vi "sum values per sequence.vi"(8 "error in":errorcluster, 11 "cycle results cluster IN":T1) -> (0 "Sequence Results":dbl[][](array[numeric]), 3 "cycle results cluster out":T1)   [LabVIEW 2016]
doc: "Takes a sample type and sorts by sequence"
uses:
  controls/cycle results control.ctl
  <vilib>/Analysis/baseanly.llb/Mean (DBL).vi
  <vilib>/Analysis/NI_AALBase.lvlib
panel:
  out "error out":errorcluster
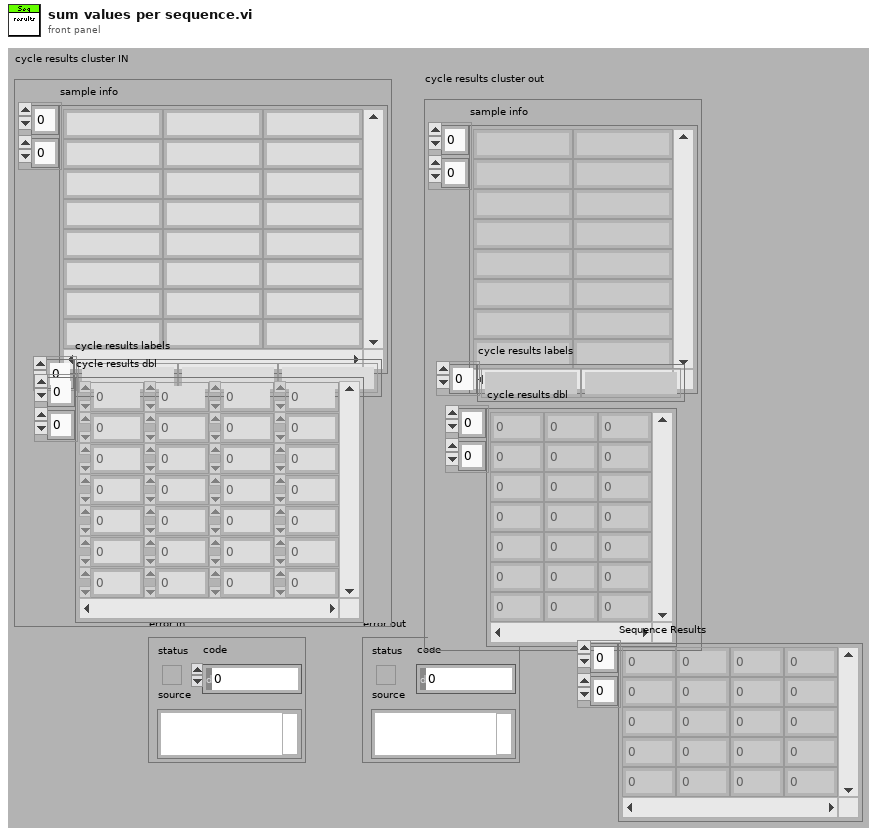
[diagram p1: front panel]
types:
  T1 = typedef "cycle results control.ctl" = cluster{"sample info":string[][], "cycle results labels":string[], "cycle results dbl":dbl[][]}
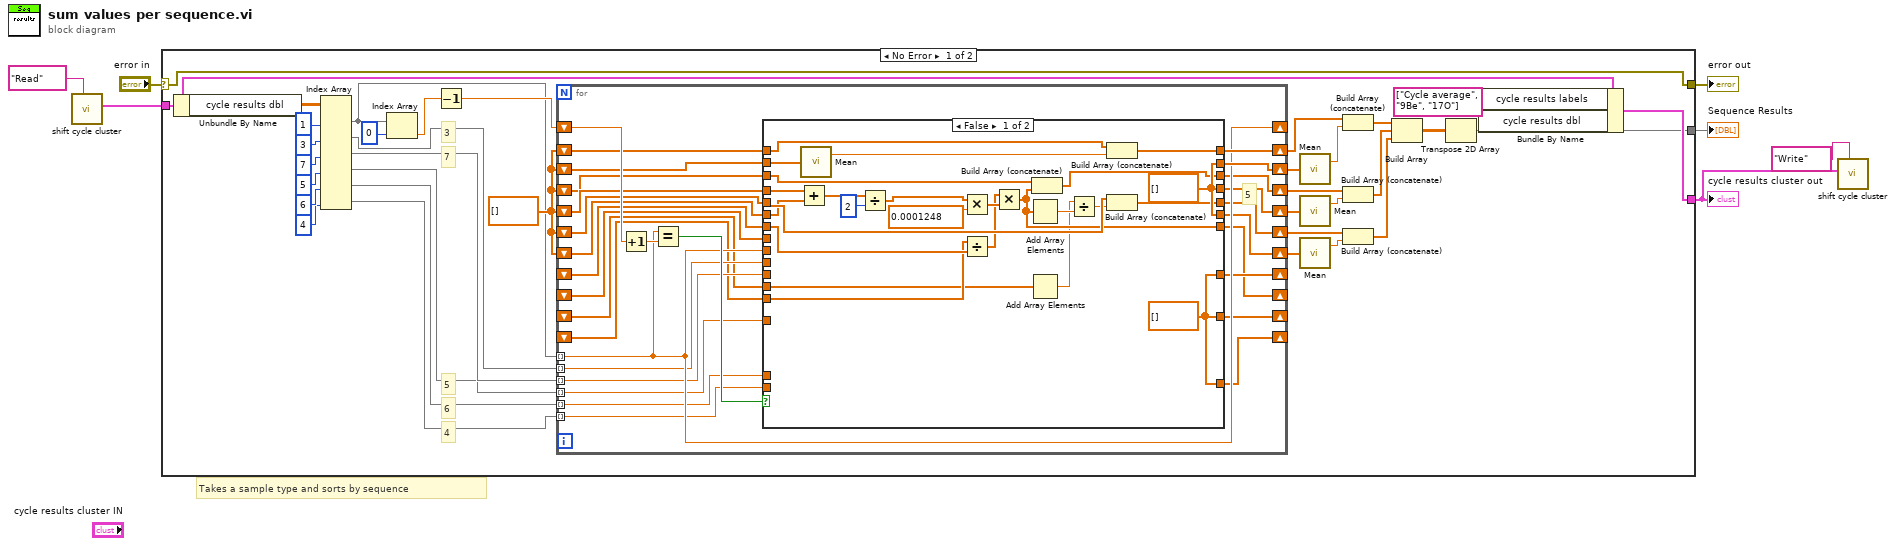
[diagram p0: block diagram]
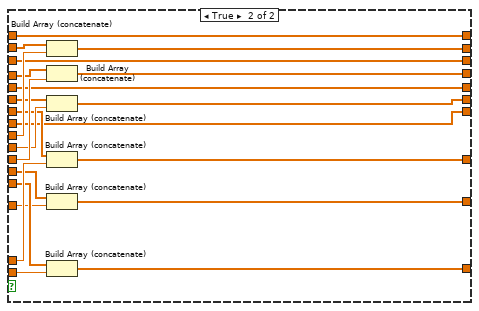
[diagram p2: hidden frame]
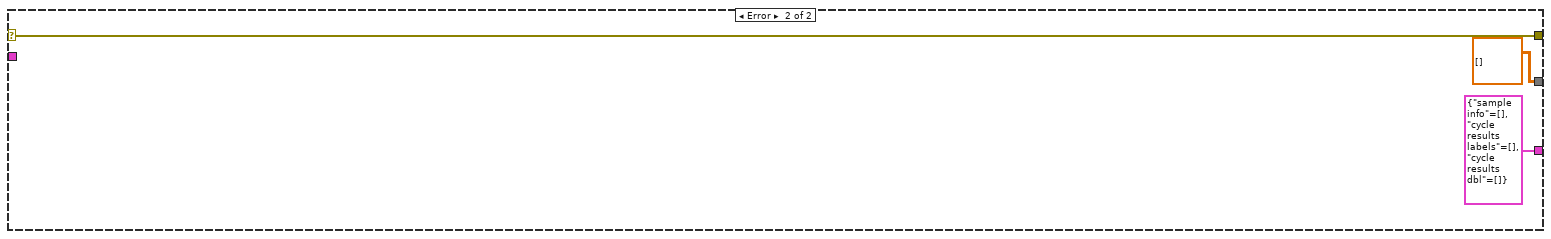
[diagram p3: hidden frame]
diagram:
  # "Takes a sample type and sorts by sequence"
  n1 = call "shift cycle cluster.vi"("read write shift"="Read") -> ("cycle results cluster out"=w3:T1)  [unwired: 9 in, 1 out]
  n2 = case shown="No Error" "error in" {
    selector: "error in" -> [w19 w120]
    tunnel: w3 -> [w18 _]
    tunnel: [w8 dbl[][] []] -> w7
    tunnel: [w16 T1 {"sample info"=[], "cycle results labels"=[], "cycle results dbl"=[]} ("cycle results cluster IN")] -> w1
    tunnel: [w19 w120] -> w5
    frame No Error {
      w32 = dbl[] []
      # "7"
      # "3"
      # "4"
      # "6"
      # "5"
      n3 = Unbundle By Name(w18) -> ("cycle results dbl"=w29:dbl[][])
      n4 = Index Array(array=w29, index (col) #1=1 ("disabled index (col)"), index (col) #2=3 ("index (col)"), index (col) #3=7 ("index (col)"), index (col) #4=5 ("index (col)"), index (col) #5=6 ("index (col)"), index (col) #6=4 ("index (col)")) -> (element #1=w25:dbl[], element #2=w24:dbl[], element #3=w23:dbl[], element #4=w12:dbl[], element #5=w11:dbl[], element #6=w10:dbl[])  [unwired: 6 in]
      n5 = Index Array(array=w25, index=0) -> (element=w33:dbl)
      n6 = Decrement(x=w33) -> (x-1=w31:dbl)
      n7 = for {
        tunnel: w25 -> [w64] mode=indexing
        shift-right: [w68] -> w35
        shift-left: w32 -> [w67]
        shift-right: [w66] -> w42
        shift-left: w32 -> [w65]
        shift-right: [w64] -> _
        shift-left: w31 -> [w71]
        tunnel: w23 -> [w63] mode=indexing
        tunnel: w24 -> [w62] mode=indexing
        shift-right: [w61] -> w34
        shift-left: w32 -> [w58]
        shift-right: [w60] -> w36
        shift-left: w32 -> [w59]
        shift-right: [w57] -> w37
        shift-left: w32 -> [w55]
        shift-right: [w56] -> w40
        shift-left: w32 -> [w54]
        tunnel: w12 -> [w45] mode=indexing
        tunnel: w11 -> [w52] mode=indexing
        tunnel: w10 -> [w53] mode=indexing
        shift-right: [w51] -> _
        shift-left: _ -> [w48]
        shift-right: [w50] -> _
        shift-left: _ -> [w49]
        shift-right: [w47] -> _
        shift-left: _ -> [w46]
        shift-right: [w44] -> _
        shift-left: _ -> [w43]
        # "5"
        n8 = Increment(x=w71) -> (x+1=w70:dbl)
        n9 = Equal?(x=w64, y=w70) -> (x = y?=w69:bool)
        n10 = case shown="False" w69 {
          tunnel: w64 -> [_ w115]
          tunnel: [w92 w118] -> w68
          tunnel: w67 -> [w96 w116]
          tunnel: [w95 w117] -> w66
          tunnel: w65 -> [w94 w117]
          tunnel: w63 -> [_ w114]
          tunnel: w62 -> [_ w113]
          tunnel: [w92 w112] -> w61
          tunnel: [w92 w111] -> w60
          tunnel: w59 -> [w87 w110]
          tunnel: w58 -> [w86 w109]
          tunnel: [w91 w108] -> w57
          tunnel: [w90 w107] -> w56
          tunnel: w55 -> [w89 w108]
          tunnel: w54 -> [w88 w107]
          tunnel: w53 -> [_ w106]
          tunnel: w52 -> [_ w105]
          tunnel: [w72 w104] -> w51
          tunnel: [w72 w103] -> w50
          tunnel: w49 -> [w80 w102]
          tunnel: w48 -> [w81 w101]
          tunnel: [w75 w100] -> w47
          tunnel: w46 -> [_ w100]
          tunnel: w45 -> [_ w99]
          tunnel: [w72 w98] -> w44
          tunnel: w43 -> [w76 w97]
          frame False {
            w72 = dbl[] []
            w92 = dbl[] []
            n11 = Add(x=w87, y=w86) -> (x+y=w82:dbl[])
            n12 = call-poly <vilib>:"Mean.vi"("X"=w96) -> ("mean"=w93:dbl)  [unwired: 1 out]
            n13 = Divide(x=w82, y=2) -> (x/y=w83:dbl[])
            n14 = Multiply(x=w83, y=0.0001248) -> (x*y=w79:dbl[])
            n15 = Divide(x=w80, y=w81) -> (x/y=w78:dbl[])
            n16 = Multiply(x=w78, y=w79) -> (x*y=w75:dbl[])
            n17 = Add Array Elements(numeric array=w75) -> (sum=w74:dbl)
            n18 = Add Array Elements(numeric array=w76) -> (sum=w73:dbl)
            n19 = Build Array (concatenate)(w89, w75) -> (w91:dbl[])
            n20 = Divide(x=w73, y=w74) -> (x/y=w77:dbl)
            n21 = Build Array (concatenate)(w94, w93) -> (w95:dbl[])
            n22 = Build Array (concatenate)(w88, w77) -> (w90:dbl[])
          }
          frame True {
            n23 = Build Array (concatenate)(w116, w115) -> (w118:dbl[])
            n24 = Build Array (concatenate)(w110, w114) -> (w111:dbl[])
            n25 = Build Array (concatenate)(w109, w113) -> (w112:dbl[])
            n26 = Build Array (concatenate)(w101, w105) -> (w104:dbl[])
            n27 = Build Array (concatenate)(w97, w99) -> (w98:dbl[])
            n28 = Build Array (concatenate)(w102, w106) -> (w103:dbl[])
          }
        }
      }
      n29 = call-poly <vilib>:"Mean.vi"("X"=w35) -> ("mean"=w41:dbl)  [unwired: 1 out]
      n30 = call-poly <vilib>:"Mean.vi"("X"=w36) -> ("mean"=w38:dbl)  [unwired: 1 out]
      n31 = call-poly <vilib>:"Mean.vi"("X"=w34) -> ("mean"=w39:dbl)  [unwired: 1 out]
      n32 = Build Array (concatenate)(w42, w41) -> (w21:dbl[])
      n33 = Build Array (concatenate)(w37, w38) -> (w22:dbl[])
      n34 = Build Array (concatenate)(w40, w39) -> (w20:dbl[])
      n35 = Build Array(w21, w22, w20) -> (w9:dbl[][])
      n36 = Transpose 2D Array(2D array=w9) -> (transposed array=w8:dbl[][])
      n37 = Bundle By Name(cluster=w18, "cycle results labels"=string[] ["Cycle average", "9Be", "17O"], "cycle results dbl"=w8) -> (w16:T1)
    }
    frame Error {
    }
  }
  "error out" <- w5
  "cycle results cluster out" <- w1
  "Sequence Results" <- w7
  n38 = call "shift cycle cluster.vi"("read write shift"="Write", "cycle results cluster In"=w1) -> ()  [unwired: 8 in, 2 out]
